vi "控速.vi"(5 "PWM1":T1, 6 "速度":dbl[](array[numeric]), 7 "PWM2":T1, 8 "错误输入（无错误）":errorcluster, 9 "DIO":T8, 10 "PWM 4":T1, 11 "PWM 3":T1) -> (0 "错误输出":errorcluster)   [LabVIEW 2016]
uses:
  <vilib>/myRIO/Instrument Drivers/Onboard IO/DIO/typedefs/DIO Reference.ctl
  <vilib>/myRIO/Common/Instrument Driver Framework/Utilities/typedefs/myRIO Generic Hardware Reference.ctl
  <vilib>/myRIO/Common/Instrument Driver Framework/Utilities/typedefs/Hardware Version Enum.ctl
  <vilib>/myRIO/Common/Instrument Driver Framework/Utilities/typedefs/myRIO v1.0 Reference.ctl
  <vilib>/myRIO/Common/Instrument Driver Framework/Utilities/typedefs/Generic FPGA Reference.ctl
  <vilib>/myRIO/Common/Instrument Driver Framework/myRIO v1.0/DIO/typedefs/DIO Channels List.ctl
  <vilib>/myRIO/Common/Instrument Driver Framework/myRIO v1.0/DIO/typedefs/DIO Channels Enum.ctl
  <vilib>/myRIO/Instrument Drivers/Onboard IO/PWM/typedefs/PWM Reference.ctl
  <vilib>/myRIO/Common/Instrument Driver Framework/myRIO v1.0/PWM/typedefs/PWM Channels Enum.ctl
  <vilib>/myRIO/Instrument Drivers/Onboard IO/PWM/typedefs/PWM Configuration.ctl
  <vilib>/Utility/error.llb/Error Cluster From Error Code.vi
  <vilib>/myRIO/Common/Instrument Driver Framework/myRIO v1.0/PWM/vis/myRIO v1.0 Write PWM.vi
  <vilib>/myRIO/Common/Instrument Driver Framework/myRIO v1.0/DIO/vis/myRIO v1.0 Write DIO.vi
  <vilib>/myRIO/Instrument Drivers/Onboard IO/PWM/PWM.lvlib
  <vilib>/myRIO/Instrument Drivers/Onboard IO/DIO/DIO.lvlib
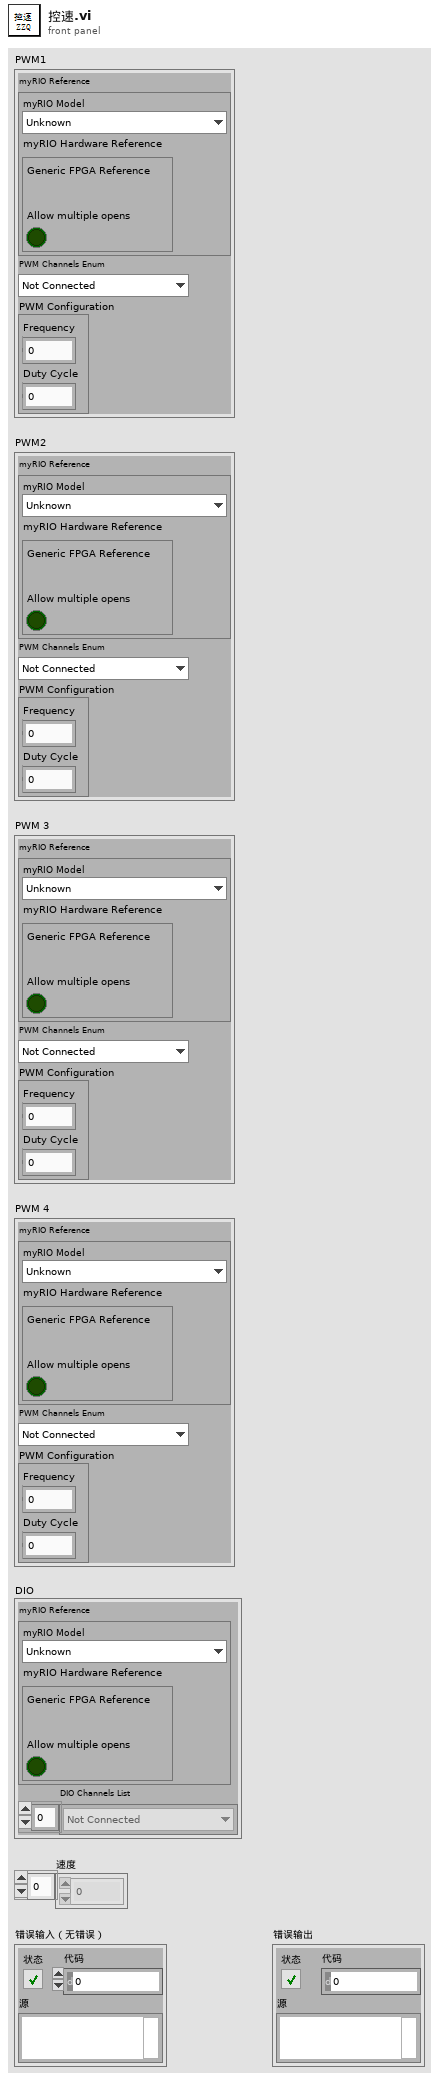
[diagram p1: front panel]
types:
  T1 = typedef "PWM.lvlib/PWM Reference.ctl" = cluster{"myRIO Reference":T2, "PWM Channels Enum":T6, "PWM Configuration":T7}
  T2 = typedef "myRIO Generic Hardware Reference.ctl" = cluster{"myRIO Model":T3, "myRIO Hardware Reference":T4}
  T3 = typedef "Hardware Version Enum.ctl" = enum16{"Unknown", "myRIO-1900", "myRIO-1950", "roboRIO", "NI ELVIS RIO CM"}
  T4 = typedef "myRIO v1.0 Reference.ctl" = cluster{"Generic FPGA Reference":T5, "Allow multiple opens":bool}
  T5 = typedef "Generic FPGA Reference.ctl" = refnum<k20>
  T6 = typedef "PWM Channels Enum.ctl" = enum16{"Not Connected", "C/PWM0", "C/PWM1", "A/PWM0", "A/PWM1", "A/PWM2", "B/PWM0", "B/PWM1", "B/PWM2", "PWM/PWM0", "PWM/PWM1", "PWM/PWM2", "PWM/PWM3", "PWM/PWM4", "PWM/PWM5", "PWM/PWM6", "PWM/PWM7", "PWM/PWM8", "PWM/PWM9"}
  T7 = typedef "PWM.lvlib/PWM Configuration.ctl" = cluster{"Frequency":dbl, "Duty Cycle":dbl}
  T8 = typedef "DIO.lvlib/DIO Reference.ctl" = cluster{"myRIO Reference":T2, "DIO Channels List":T9}
  T9 = typedef "DIO Channels List.ctl" = T10[]
  T10 = typedef "DIO Channels Enum.ctl" = enum16{"Not Connected", "C/DIO0", "C/DIO1", "C/DIO2", "C/DIO3", "C/DIO4", "C/DIO5", "C/DIO6", "C/DIO7", "A/DIO0", "A/DIO1", "A/DIO2", "A/DIO3", "A/DIO4", "A/DIO5", "A/DIO6", "A/DIO7", "A/DIO8", "A/DIO9", "A/DIO10", "A/DIO11", "A/DIO12", "A/DIO13", "A/DIO14", "A/DIO15", "B/DIO0", "B/DIO1", "B/DIO2", "B/DIO3", "B/DIO4", "B/DIO5", "B/DIO6", "B/DIO7", "B/DIO8", "B/DIO9", "B/DIO10", "B/DIO11", "B/DIO12", "B/DIO13", "B/DIO14", "B/DIO15", "LED0", "LED1", "LED2", "LED3", "Button0", "DIO/DIO0", "DIO/DIO1", "DIO/DIO2", "DIO/DIO3", "DIO/DIO4", "DIO/DIO5", "DIO/DIO6", "DIO/DIO7", "DIO/DIO8", "DIO/DIO9", "SPI/CS0", "SPI/CS1", "SPI/CS2", "SPI/CS3", "LED RADIO (Green)", "LED RADIO (Red)", "LED COMM (Green)", "LED COMM (Red)", "LED MODE (Green)", "LED MODE (Red)"}
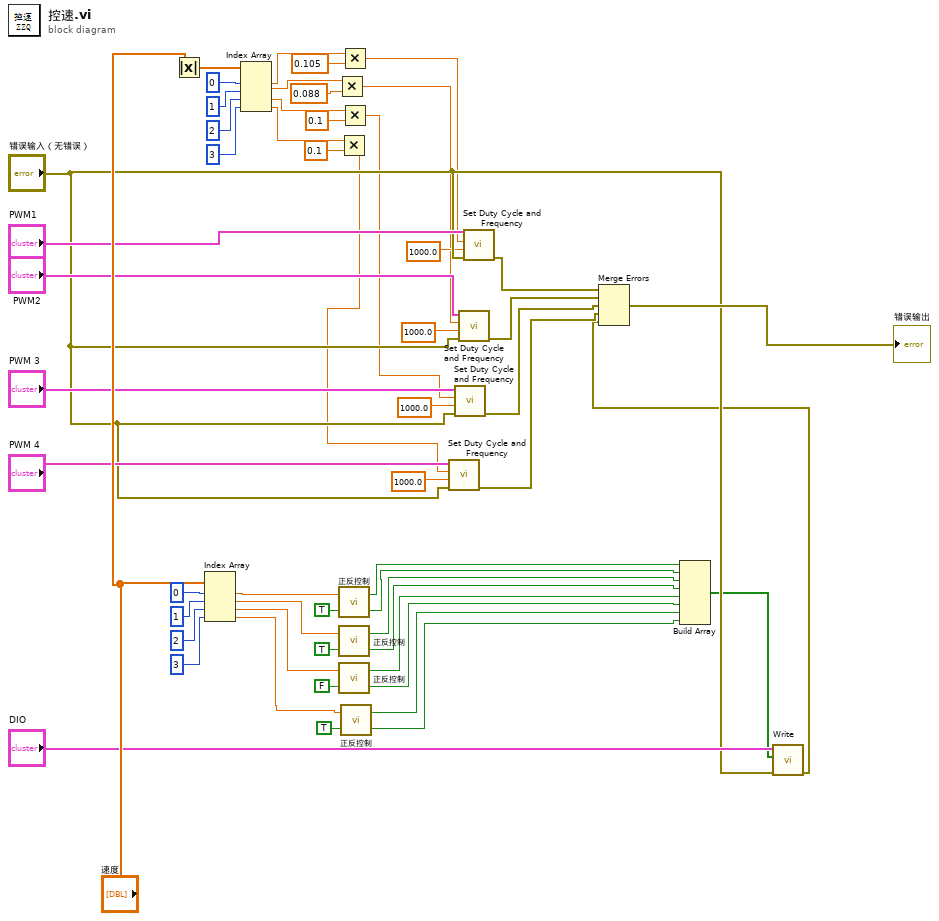
[diagram p0: block diagram]
diagram:
  n1 = Absolute Value(x="速度") -> (abs(x)=w27:dbl[])
  n2 = Index Array(array="速度", index #1=0 ("索引"), index #2=1 ("索引"), index #3=2 ("索引"), index #4=3 ("索引")) -> (element #1=w18:dbl, element #2=w13:dbl, element #3=w12:dbl, element #4=w11:dbl)
  n3 = Index Array(array=w27, index #1=0 ("索引"), index #2=1 ("索引"), index #3=2 ("索引"), index #4=3 ("索引")) -> (element #1=w35:dbl, element #2=w34:dbl, element #3=w33:dbl, element #4=w32:dbl)
  n4 = Multiply(x=w34, y=0.088) -> (x*y=w25:dbl)
  n5 = Multiply(x=w32, y=0.1) -> (x*y=w23:dbl)
  n6 = call "正反控制.vi"("接法"=TRUE, "x"=w18) -> ("INB"=w8:bool, "INA"=w9:bool)
  n7 = call "正反控制.vi"("接法"=TRUE, "x"=w13) -> ("INB"=w6:bool, "INA"=w7:bool)
  n8 = call "正反控制.vi"("接法"=FALSE, "x"=w12) -> ("INB"=w4:bool, "INA"=w5:bool)
  n9 = Multiply(x=w35, y=0.105) -> (x*y=w26:dbl)
  n10 = Multiply(x=w33, y=0.1) -> (x*y=w24:dbl)
  n11 = call "正反控制.vi"("接法"=TRUE, "x"=w11) -> ("INB"=w2:bool, "INA"=w3:bool)
  n12 = call <vilib>:"Set Duty Cycle and Frequency.vi"("error in (no error)"="错误输入（无错误）", "Frequency [Hz]"=1000.0, "Duty Cycle"=w23, "PWM Ref In"="PWM 4") -> ("error out"=w40:errorcluster)  [unwired: 5 in, 1 out]
  n13 = call <vilib>:"Set Duty Cycle and Frequency.vi"("error in (no error)"="错误输入（无错误）", "Frequency [Hz]"=1000.0, "Duty Cycle"=w24, "PWM Ref In"="PWM 3") -> ("error out"=w41:errorcluster)  [unwired: 5 in, 1 out]
  n14 = call <vilib>:"Set Duty Cycle and Frequency.vi"("error in (no error)"="错误输入（无错误）", "Frequency [Hz]"=1000.0, "Duty Cycle"=w25, "PWM Ref In"="PWM2") -> ("error out"=w42:errorcluster)  [unwired: 5 in, 1 out]
  n15 = call <vilib>:"Set Duty Cycle and Frequency.vi"("error in (no error)"="错误输入（无错误）", "Frequency [Hz]"=1000.0, "Duty Cycle"=w26, "PWM Ref In"="PWM1") -> ("error out"=w43:errorcluster)  [unwired: 5 in, 1 out]
  n16 = Build Array(w9, w8, w7, w6, w5, w4, w3, w2) -> (w10:bool[])
  n17 = call <vilib>:"Write.vi"("error in (no error)"="错误输入（无错误）", "Values"=w10, "DIO Ref In"="DIO") -> ("error out"=w1:errorcluster)  [unwired: 6 in, 1 out]
  n18 = Merge Errors(w43, w42, w41, w40, w1) -> (→"错误输出":errorcluster)
